vi "Place Elves.vi"(10 "Elf Locations":T1[](array[typedef]), 11 "Spaced Grove in":T2[][](array[typedef])) -> (3 "Spaced Grove out":T2[][](array[typedef]))   [LabVIEW 2023]
uses:
  RB ENUM_Spot ID.ctl
  Cluster _Point Location.ctl
  e5b75d54-041b-471f-b42f-310e9ff871b2.vi
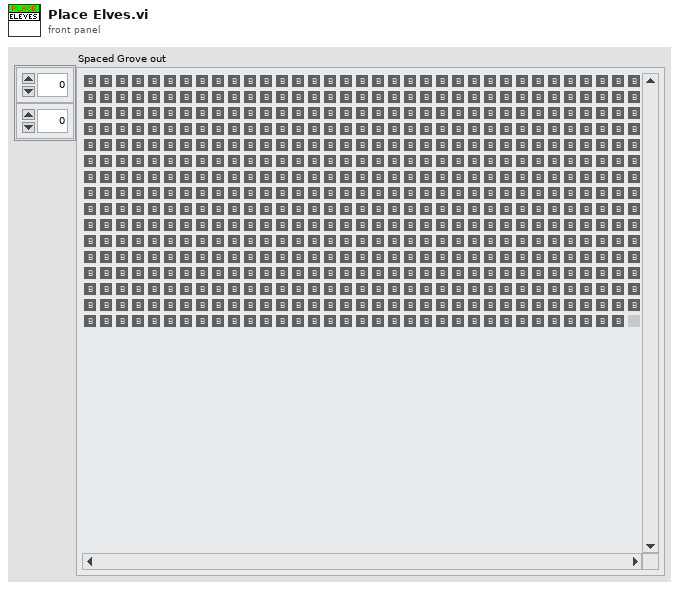
[diagram p1: front panel]
types:
  T1 = typedef "Cluster _Point Location.ctl" = cluster{"X col":i32, "Y row":i32}
  T2 = typedef "RB ENUM_Spot ID.ctl" = enum32{"Blank", "ELF", "Proposed"}
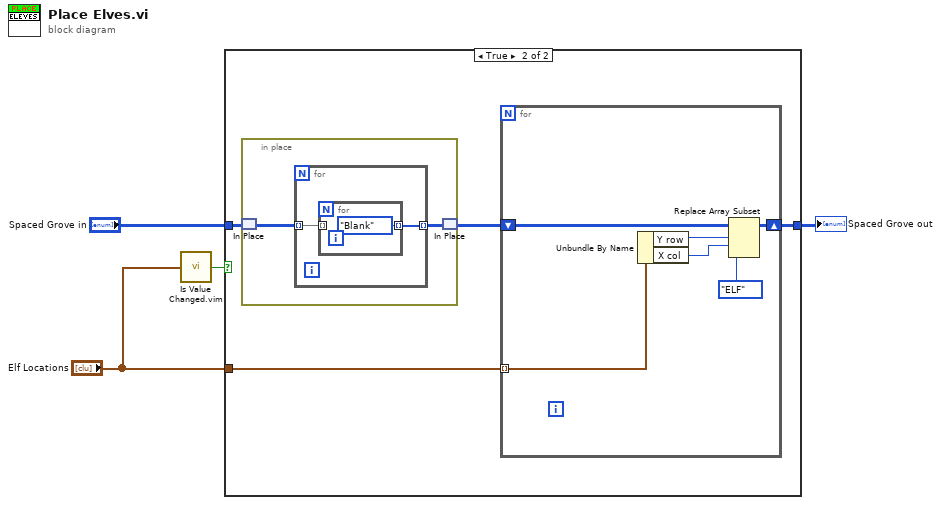
[diagram p0: block diagram]
diagram:
  n1 = call "Is Value Changed.vim"("value"="Elf Locations") -> ("changed or first call?"=w1:bool)
  n2 = case shown="True" w1 {
    tunnel: "Spaced Grove in" -> [w5 w9]
    tunnel: [w5 w7] -> w3
    tunnel: "Elf Locations" -> [_ w6]
    frame False {
    }
    frame True {
      n3 = in-place {
        n4 = in-place-match #1(w9) -> (w17:T2[][])
        n5 = for {
          tunnel: w17 -> [w19] mode=indexing
          tunnel: [w18] -> w16 mode=indexing
          n6 = for {
            tunnel: w19 -> [_] mode=indexing
            tunnel: [RB_ENUM_Spot_ID."Blank" ("Spot")] -> w18 mode=indexing
          }
        }
        n7 = in-place-match #1(w16) -> (w8:T2[][])
      }
      n8 = for {
        shift-right: [w14] -> w7
        shift-left: w8 -> [w15]
        tunnel: w6 -> [w10] mode=indexing
        n9 = Unbundle By Name(w10) -> ("Y row"=w12:i32, "X col"=w11:i32)
        n10 = Replace Array Subset(array=w15, new element=RB_ENUM_Spot_ID."ELF" ("Spot"), index (row)=w12, index (col)=w11) -> (w14:T2[][])
      }
    }
  }
  "Spaced Grove out" <- w3
